vi "VariantClusterAccess.vi"(8 "error in (no error)":errorcluster, 9 "label":string, 10 "index":i32=-1, 11 "Cluster Variable":variant) -> (0 "error out":errorcluster, 1 "rest":string, 2 "value":variant, 3 "prepend":string, 5 "type string":i16[](array[numeric]))   [LabVIEW 2020]
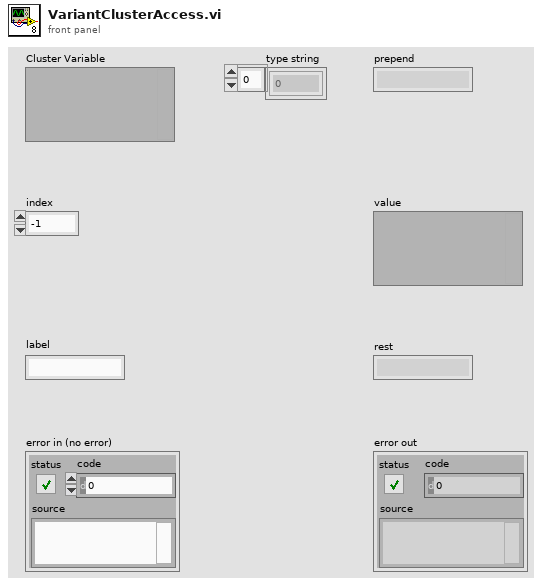
[diagram p1: front panel]
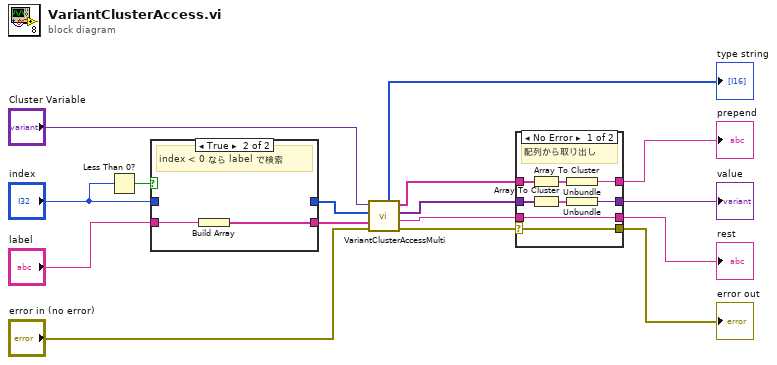
[diagram p0: block diagram]
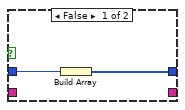
[diagram p3: hidden frame]
diagram:
  n1 = Less Than 0?(x="index") -> (x < 0?=w16:bool)
  n2 = case shown="True" w16 {
    tunnel: "label" -> [_ w20]
    tunnel: "index" -> [w18 _]
    tunnel: [_ w19] -> w12
    tunnel: [w17 _] -> w13
    frame False {
      n3 = Build Array(w18) -> (w17:i32[])
    }
    frame True {
      # "index < 0 なら label で検索"
      n4 = Build Array(w20) -> (w19:string[])
    }
  }
  n5 = call "VariantClusterAccessMulti.vi"("error in (no error)"="error in (no error)", "labels"=w12, "indices"=w13, "Value in"="Cluster Variable") -> ("error out"=w9:errorcluster, "rest"=w7:string, "values"=w5:variant[], "prepends"=w4:string[], "type string"=→"type string":i16[])  [unwired: 3 in]
  n6 = case shown="No Error" w9 {
    selector: w9 -> [w28 w29]
    tunnel: [w28 w29] -> w8
    tunnel: [w27 _] -> w6
    tunnel: w7 -> [w27 _]
    tunnel: w5 -> [w26 _]
    tunnel: w4 -> [w23 _]
    tunnel: [w22 _] -> w2
    tunnel: [w21 _] -> w1
    frame No Error {
      # "配列から取り出し"
      n7 = Array To Cluster(array=w23) -> (cluster=w24:cluster{"prepends[0]":string})
      n8 = Array To Cluster(array=w26) -> (cluster=w25:cluster{"values[0]":variant})
      n9 = Unbundle(w24) -> ("prepends[0]"=w22:string)
      n10 = Unbundle(w25) -> ("values[0]"=w21:variant)
    }
    frame Error {
    }
  }
  "error out" <- w8
  "rest" <- w6
  "prepend" <- w2
  "value" <- w1
